vi "Show With Fade In.vi"(8 "error in (no error)":errorcluster, 9 "Target Transparency (0)":u8, 10 "Fade time (800ms)":i32=800, 11 "Philips Dialog in":refnum<class "Flex UI Dialog.lvclass">) -> (0 "error out":errorcluster, 3 "Philips Dialog out":refnum<class "Flex UI Dialog.lvclass">)   [LabVIEW 2014, in "Flex UI Dialog.lvclass"]
doc: "Display the UI with a fade in time and transparency level."
uses:
  Flex UI Dialog.lvclass
  <vilib>/LAVA/UI Tools/Fading/_fadetype__lava_lib_ui_tools.ctl
  Flex UI (Parent)/Flex UI.lvclass/Flex UI.ctl
  <vilib>/LAVA/UI Tools/Fading/_Fade(I32)__lava_lib_ui_tools.vi
  Flex UI (Parent)/Flex UI.lvclass
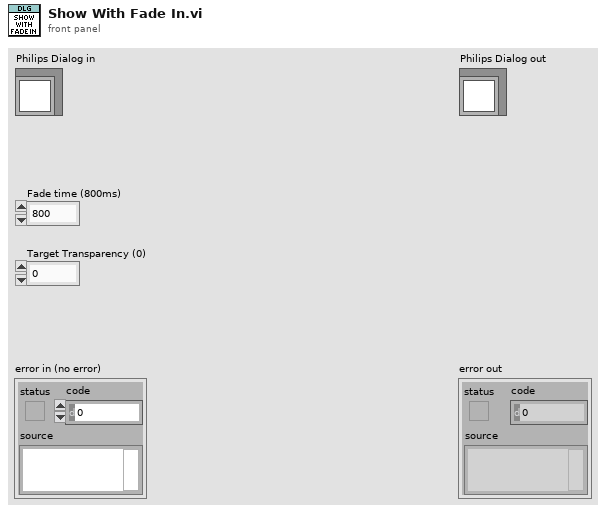
[diagram p1: front panel]
types:
  T1 = typedef "_fadetype__lava_lib_ui_tools.ctl" = enum16{"Exponential", "Linear"}
  T2 = enum32{"Invalid", "Standard", "Closed", "Hidden", "Minimized", "Maximized"}
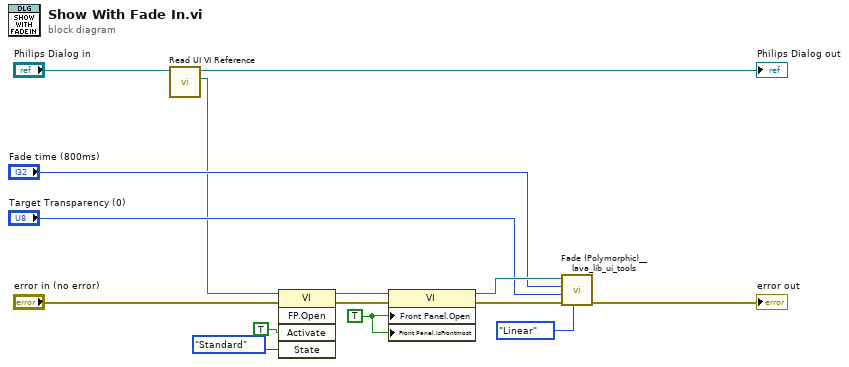
[diagram p0: block diagram]
diagram:
  w2 = TRUE ("Front Panel Window:Open")
  n1 = call "Read UI VI Reference.vi"("Philips UI in"="Philips Dialog in") -> ("UI VI Reference"=w5:refnum<vi>, "Philips UI out"=→"Philips Dialog out":refnum<class "Flex UI Dialog.lvclass">)  [unwired: 9 in]
  n2 = invoke class="VI" method="FP.Open"(reference=w5, error in="error in (no error)", "Activate"=TRUE ("Activate?"), "State"=T2."Standard") -> (reference out=w3:refnum<vi>, error out=w4:errorcluster)  [unwired: 1 in, 3 out]
  n3 = property class="VI"(reference=w3, error in=w4, "Front Panel.Open"=w2, "Front Panel.IsFrontmost"=w2) -> (reference out=w12:refnum<vi>, error out=w13:errorcluster)
  n4 = call-poly <vilib>:"Fade (Polymorphic)__lava_lib_ui_tools.vi"("Fade (Exponential)"=_fadetype__lava_lib_ui_tools."Linear", "error in"=w13, "Target Transparency (0)"="Target Transparency (0)", "Fade time (ms)"="Fade time (800ms)", "VI Reference (calling VI)"=w12) -> ("error out"=→"error out":errorcluster)  [unwired: 5 in, 1 out]
